vi "Read Use System Alert_.vi"(8 "error in (no error)":errorcluster, 11 "Write Beep Parameters Msg in":refnum<class "Write Beep Parameters Msg.lvclass">) -> (0 "error out":errorcluster, 2 "Use System Alert?":bool, 3 "Write Beep Parameters Msg out":refnum<class "Write Beep Parameters Msg.lvclass">)   [LabVIEW 2016, in "CS++BeepActor.lvlib" / "Write Beep Parameters Msg.lvclass"]
uses:
  Write Beep Parameters Msg.lvclass
  Write Beep Parameters Msg.lvclass/Write Beep Parameters Msg.ctl
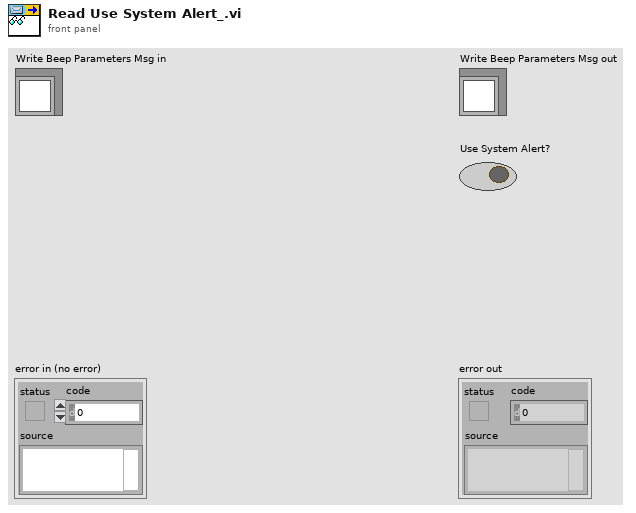
[diagram p1: front panel]
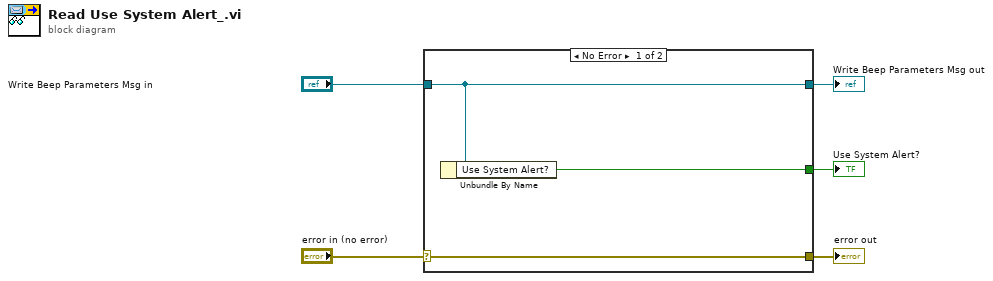
[diagram p0: block diagram]
diagram:
  n1 = case shown="No Error" "error in (no error)" {
    selector: "error in (no error)" -> [w8 w9]
    tunnel: [w8 w9] -> w4
    tunnel: [w7 w10] -> w2
    tunnel: "Write Beep Parameters Msg in" -> [w7 w10]
    tunnel: [w6 _] -> w1
    frame No Error {
      n2 = Unbundle By Name(w7) -> ("Use System Alert?"=w6:bool)
    }
    frame Error {
    }
  }
  "error out" <- w4
  "Write Beep Parameters Msg out" <- w2
  "Use System Alert?" <- w1
